vi "Extract Ollama Response.vi"(0 "headers":string, 5 "body":string, 11 "error in":errorcluster) -> (4 "value":string, 15 "error out":errorcluster)   [LabVIEW 2020, in "llm_ollama_chatmodels.lvclass"]
uses:
  llm_ollama_chatmodels.lvclass
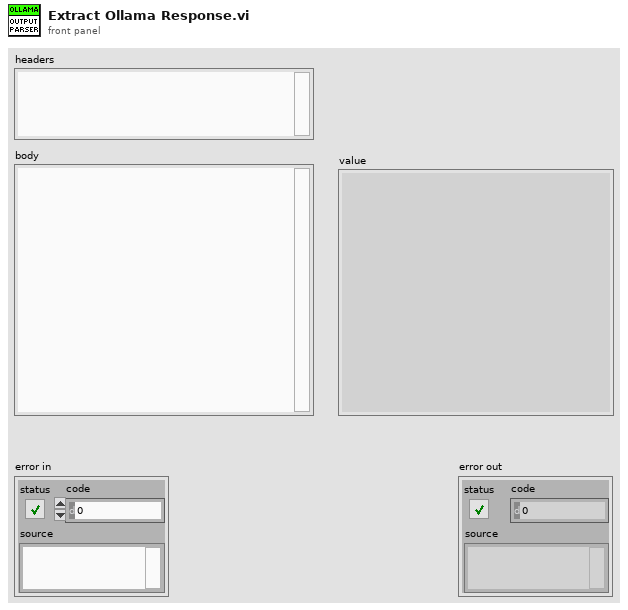
[diagram p1: front panel]
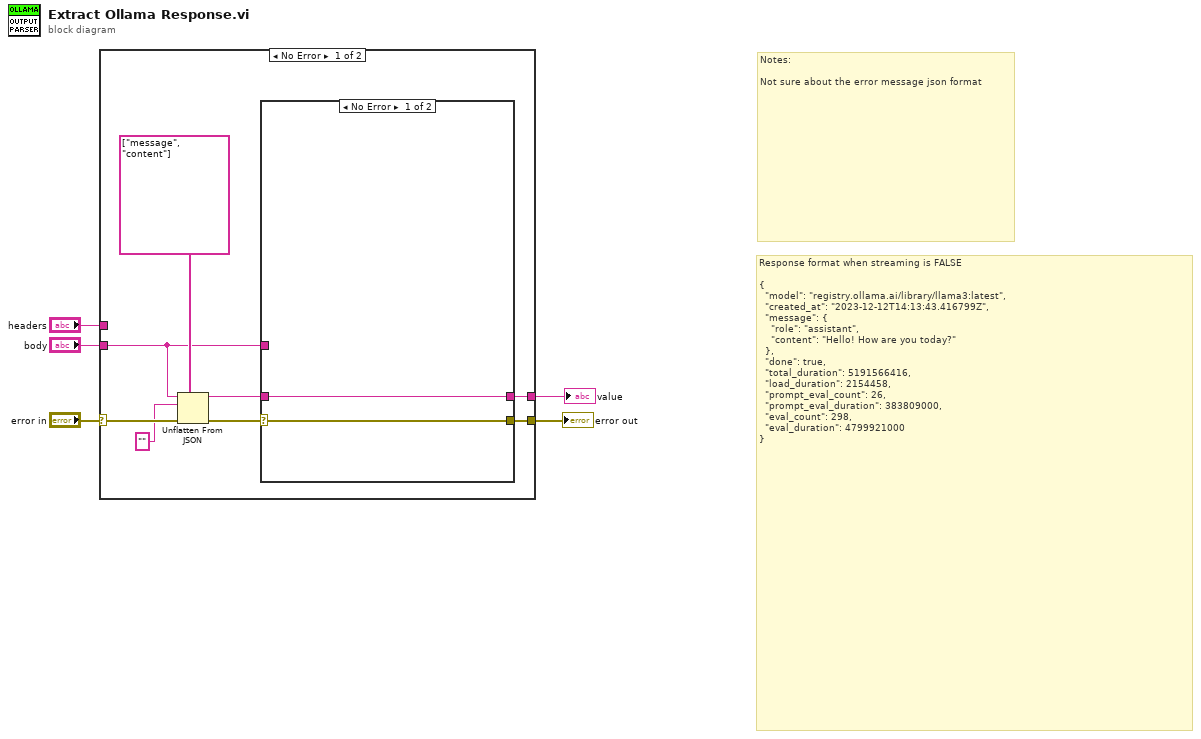
[diagram p0: block diagram]
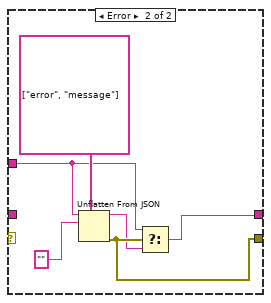
[diagram p2: hidden frame]
diagram:
  # "Response format when streaming is FALSE\n\n{\n  \"model\": \"registry.ollama.ai/library/llama3:latest\",\n  \"created_at\": \"2023-12-12T14:13:43.416799Z\",\n  \"message\": {\n    \"role\": \"assistant\",\n    \"content\": \"Hello! How are you today?\"\n  },\n  \"done\": true,\n  \"total_duration\": 5191566416,\n  \"load_duration\": 2154458,\n  \"prompt_eval_count\": 26,\n  \"prompt_eval_duration\": 383809000,\n  \"eval_count\": 298,\n  \"eval_duration\": 4799921000\n}"
  # "Notes:\n\nNot sure about the error message json format"
  n1 = case shown="No Error" "error in" {
    selector: "error in" -> [w13 w23]
    tunnel: [w9 w23] -> w4
    tunnel: "body" -> [w8 _]
    tunnel: "headers" -> [_ w22]
    tunnel: [w6 w22] -> w1
    frame No Error {
      n2 = Unflatten From JSON(path=string[] ["message", "content"], JSON string=w8, type and defaults="", error in (no error)=w13) -> (value=w7:string, error out=w10:errorcluster)  [unwired: 3 in]
      n3 = case shown="No Error" w10 {
        selector: w10 -> [w15 _]
        tunnel: [w15 w18] -> w9
        tunnel: w8 -> [_ w16]
        tunnel: w7 -> [w14 _]
        tunnel: [w14 w19] -> w6
        frame No Error {
        }
        frame Error {
          n4 = Unflatten From JSON(path=string[] ["error", "message"], JSON string=w16, type and defaults="") -> (value=w17:string, error out=w18:errorcluster)  [unwired: 4 in]
          n5 = Select(t=w16, s=w18, f=w17) -> (s? t:f=w19:string)
        }
      }
    }
    frame Error {
    }
  }
  "error out" <- w4
  "value" <- w1
